vi "Dashboard Main.vi"() -> ()   [LabVIEW 2014]
uses:
  <vilib>/event_ctls.llb/eventvkey.ctl
  <vilib>/Rock Robotics/WPI/Dashboard/WPI_DashboardLogging Global.vi
  <vilib>/Rock Robotics/Network Tables/SD Read Boolean.vi
  <vilib>/Rock Robotics/Network Tables/SD Read Number.vi
  <vilib>/Utility/config.llb/Write Key (String).vi
  <vilib>/Utility/config.llb/Write Key (I32).vi
  <vilib>/Utility/config.llb/NI_LVConfig.lvlib
panel:
  in  "TCP":refnum<k5>
  in  "Rec Mode":enum32{"Stop", "Record", "Playback"}(radio)
  in  "Vision":u16(ring) items=["Camera Off", "USB Camera SW", "USB Camera HW", "IP Camera"]
  out "Camera IP":string
  out "Image Message":string="Timeout in Camera Communications"
  in  "Dashboard Tab":T1(tab)
  in  "Camera Settings":T2={"Frame Rate"=30, "Compression"=30, "Size"=1} {"Frame Rate" scale=1.0..30.0; "Size" items=["640x480", "320x240", "160x120"]}
  out "MotorChart R":cluster{"Numeric":dbl, "Numeric":dbl}(graph)
  out "MotorChart L":T3(graph)
  out "MotorSliders R":cluster{"MotorSlide1":dbl, "MotorSlide2":dbl} {"MotorSlide2" scale=-1.0..1.0 scale format="%#_2e"; "MotorSlide1" scale=-1.0..1.0 scale format="%#_2e"}
  out "MotorSliders L":T4 {"MotorSlide4 2" scale=0.0..14.0 scale format="%#_2e"; "MotorSlide2" scale=-1.0..1.0 scale format="%#_2e"; "MotorSlide1" scale=-1.0..1.0 scale format="%#_2e"}
  out "Gyro":dbl(knob) scale=0.0..360.0
  out "JS1 Z":dbl(slide) scale=-1.0..1.0 scale format="%#_2e"
  out "JS1 Graph":cluster{"X":dbl, "Y":dbl}[](graph)
  out "JS1 Buttons":T5
  out "JS2 Z":dbl(slide) scale=-1.0..1.0 scale format="%#_2e"
  out "JS2 Graph":cluster{"X":dbl, "Y":dbl}[](graph)
  out "JS2 Buttons":T5
  out "Mode":T6(ring)=enum."Auto Disabled"
  in  "DB Camera Config":bool
  out "fps":dbl format="%#.1g"
  out "Mbps":dbl format="%#.1g"
  out "Mbps 2":bool
  in  "DB/String 9":string
  in  "DB/String 8":string
  in  "DB/String 7":string
  in  "DB/String 6":string
  in  "DB/String 5":string
  in  "DB/String 4":string
  in  "DB/String 3":string
  in  "DB/String 2":string
  in  "DB/String 1":string
  in  "DB/String 0":string
  in  "DB/Slider 0":dbl(slide) scale=0.0..5.0
  in  "DB/Slider 1":dbl(slide) scale=0.0..5.0
  in  "DB/Slider 2":dbl(slide) scale=0.0..5.0
  in  "DB/Slider 3":dbl(slide) scale=0.0..5.0
  out "DB/LED 3":bool
  out "DB/LED 2":bool
  out "DB/LED 1":bool
  out "DB/LED 0":bool
  in  "DB/Button 3":bool
  in  "DB/Button 2":bool
  in  "DB/Button 1":bool
  in  "DB/Button 0":bool caption="New Name"
  out "Lifting Arm Mode":bool
  out "Lifting Arm Direction":bool
  out "Lifting Motor Speed":dbl(knob) scale=-1.0..1.0
  out "Lower Switch":bool
  out "Upper Switch":bool
  out "Auto 3":bool
  out "Auto 2":bool
  out "Auto 4":bool
  out "Auto 1":bool
  out "Lifting Arm Running":bool
  out "Trigger Switch Activated":bool
  out "Stopper Motor Speed":dbl(knob) scale=-1.0..1.0
  in  "Test Slider":dbl(slide) scale=0.0..100.0 scale format="%#_3g"
  in  "On/Off":bool caption="Solenoid"
  in  "Test Name":u16(ring) items=["Select the test to run...", "Example Test", "-------------------------------", "List of tests is built in robot code.", "Replace with your own automated tests."]
  in  "Test Tree":string(tree)
  in  "Motor":cluster{"Value":dbl, "Enable":bool} {"Value" scale=-1.0..1.0 scale format="%#_3g"}
  out "Progress":T7 {"Test Progress" scale=0.0..100.0}
  in  "Rev/Fwd":cluster{"Forward":bool, "Reverse":bool}
  in  "Test Ring":u16(ring) items=["Monochrome", "Color"]
  in  "Listbox":i32(listbox)
  out "Tree":string(tree)
  out "Camera Image":T8(plugin-control)
  out "Boolean":bool
  # "Left"
  # "Front"
  # "Right"
  # "Battery"
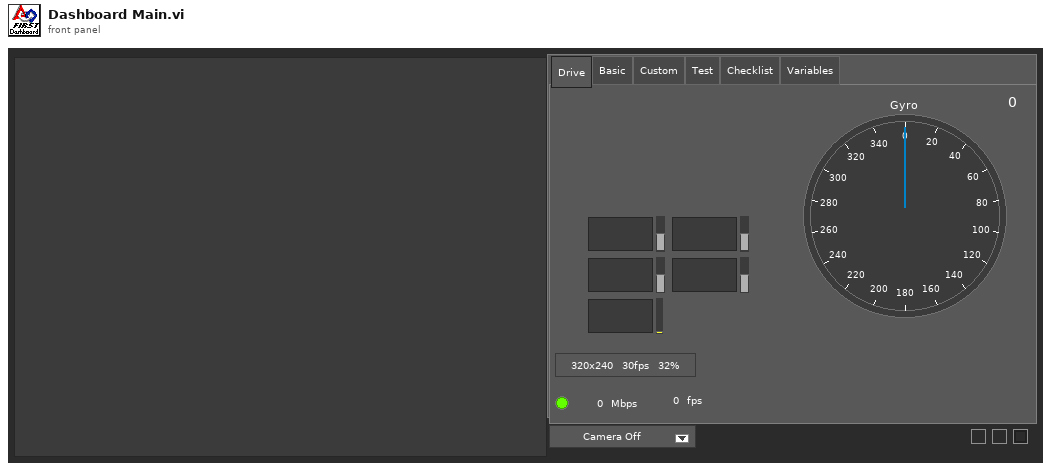
[diagram p1: front panel]
types:
  T1 = enum32{"Drive", "Basic", "Custom", "Test", "Checklist", "Variables"}
  T2 = cluster{"Frame Rate":i32, "Compression":i32, "Size":u16}
  T3 = cluster{"Numeric":dbl, "Numeric":dbl, "Battery V":dbl}
  T4 = cluster{"MotorSlide1":dbl, "MotorSlide2":dbl, "MotorSlide4 2":dbl}
  T5 = cluster{bool, bool, bool, bool, bool, bool, bool, bool, bool, bool, bool, bool}
  T6 = enum8{"Tele-Op Disabled", "Tele-Op Enabled", "Auto Disabled", "Auto Enabled", "Test Disabled", "Test Enabled", "Disconnected", "No Code", "E-Stop"}
  T7 = cluster{"Test Progress":u8, "Test Progress Text":string}
  T8 = typedef "IMAQ Image.ctl" = refnum<image>
  T9 = typedef "Image Type" = u32
  T10 = cluster{"Camera Image":refnum<vi>, "Dashboard Tab":refnum<vi>, "Boolean":refnum<vi>, "Vision":refnum<vi>, "Rec Mode":refnum<vi>, "Test Slider":refnum<vi>, "On/Off ":refnum<vi>, "Test Ring":refnum<vi>, "Rev/Fwd":refnum<vi>, "Test Name":refnum<vi>, "Motor":refnum<vi>, "Progress":refnum<vi>, "CheckList":refnum<vi>, "Tree":refnum<vi>, "Test Tree":refnum<vi>}
  T11 = cluster{"Error Strings":string, "Disable Counts":cluster{u16, u16}, "Rail Faults":cluster{u16, u16, u16}, "Robot IP":string, "DB Mode":u8, "Event Info":cluster{"Name":string, "Type":u8, "Number":u16, "Replay":u8}, "Camera Addr":string}
  T12 = cluster{"Storage":cluster{"Disk Free":u64, "RAM Block":u32, "RAM free":u32}, "CPU Utilization":cluster{"CPU % ISR":sgl, "CPU % Time Crit":sgl, "CPU % Timed Str":sgl, "CPU % High":sgl, "CPU % Above":sgl, "CPU % Normal":sgl, "CPU % Low":sgl}, "CAN":cluster{"% Bus Utilization":sgl, "Bus Off Cnt":u32, "TX_FIFO Full Cnt":u32, "Receive Error Cnt":u8, "Transmit Error Cnt":u8}, "HID":cluster{"HID Outputs":u32, "Rumble Low":u16, "Rumble High":u16}[]}
  T13 = cluster{"Status bits":cluster{"Test Mode":bool, "Autonomous":bool, "Enabled":bool, "Code Start":bool, "Brownout":bool, "Reserved 2":bool, "Reserved 3":bool, "E-Stop":bool}, "Code Trace":cluster{"Disabled":bool, "TeleOp":bool, "Auto":bool, "Test":bool}, "Controller Type":enum16{"unknown", "cRIO", "roboRio"}, "Code?":enum16{"unknown", "noCode", "code"}, "Battery V":dbl}
  T14 = cluster{"Control Bits":cluster{"TestMode":bool, "Autonomous":bool, "Enabled":bool, "FMS Present":bool, bool, bool, bool, "E-Stop":bool}, "Team Station ":u8, "Countdown":sgl, "Joystick Values":cluster{"Axes":dbl[], "Buttons":bool[], "POVs":i16[]}[]}
  T15 = cluster{"Axes":dbl[], "Buttons":bool[], "POVs":i16[]}[]
  T16 = cluster{"Axes":dbl[], "Buttons":bool[], "POVs":i16[]}
  T17 = cluster{"Buttons[0]":bool, "Buttons[1]":bool, "Buttons[2]":bool, "Buttons[3]":bool, "Buttons[4]":bool, "Buttons[5]":bool, "Buttons[6]":bool, "Buttons[7]":bool, "Buttons[8]":bool, "Buttons[9]":bool, "Buttons[10]":bool, "Buttons[11]":bool}
  T18 = typedef "NI_LVConfig.lvlib/Config Data RefNum.ctl" = refnum<k1>
  T19 = cluster{"Operation":enum16{"Update", "Clear"}, "Color Box":u32}[]
  T20 = typedef "eventvkey.ctl" = enum16{"ASCII", "Enter", "Return", "Shift", "Ctrl", "Alt", "Cmd", "Opt", "Caps", "NumLock", "Clear", "Break", "Up", "Down", "Left", "Right", "Insert", "Delete", "Home", "End", "PageUp", "PageDown", "Escape", "Help", "Pause", "ScrollLock", "F1", "F2", "F3", "F4", "F5", "F6", "F7", "F8", "F9", "F10", "F11", "F12", "F13", "F14", "F15", "F16", "F17", "F18", "F19", "F20", "F21", "F22", "F23", "F24", "Play", "VolumeUp", "VolumeDown", "Mute", "Two Byte Char"}
  T21 = cluster{"Image Size":bool, "Image Type":bool, "Pixel Value":bool, "ROI Information":bool, "Zoom Factor":bool}
  T22 = enum8{"Enabled", "Disabled", "Disabled and Grayed Out"}
  T23 = cluster{"Operation":enum16{"Update", "Clear"}, "Color Box":u32}
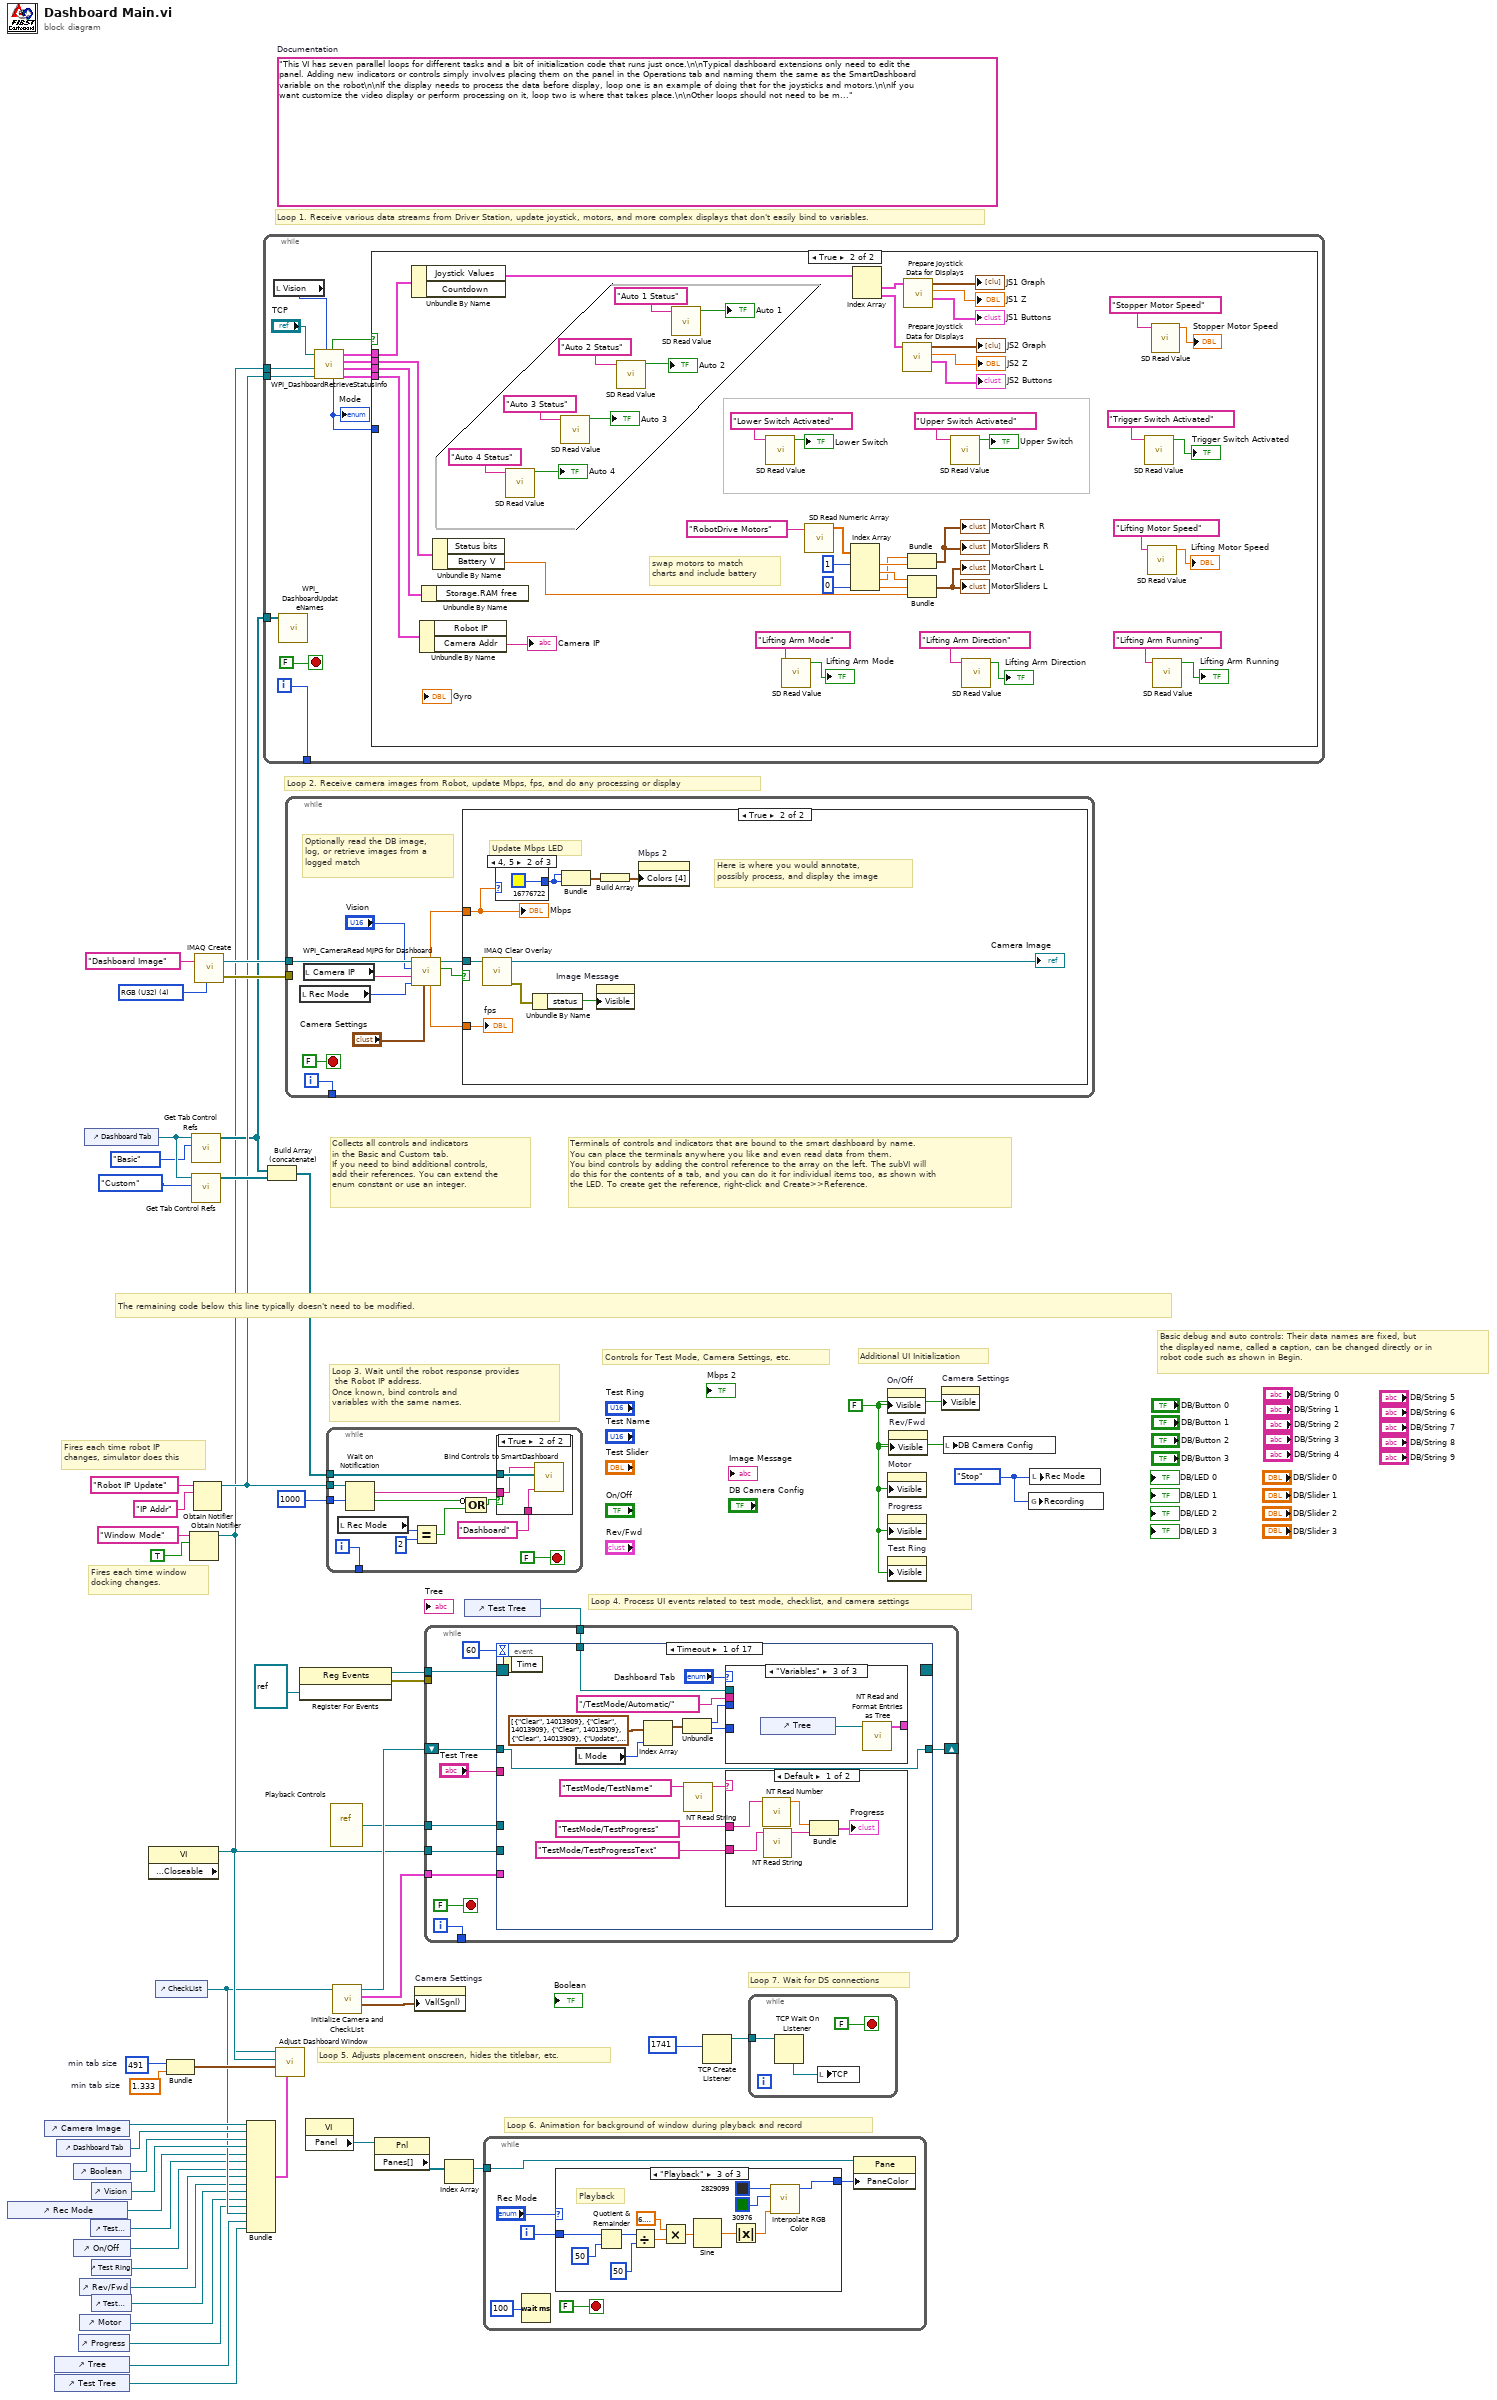
[diagram p0: block diagram]
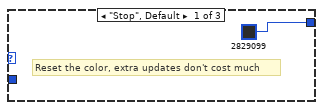
[diagram p3: hidden frame]
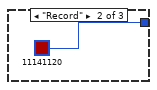
[diagram p4: hidden frame]
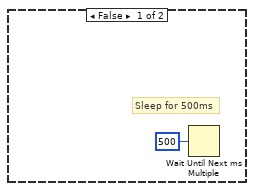
[diagram p6: hidden frame]
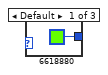
[diagram p7: hidden frame]
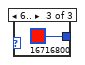
[diagram p8: hidden frame]
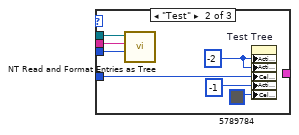
[diagram p10: hidden frame]
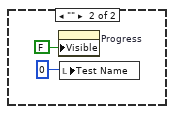
[diagram p11: hidden frame]
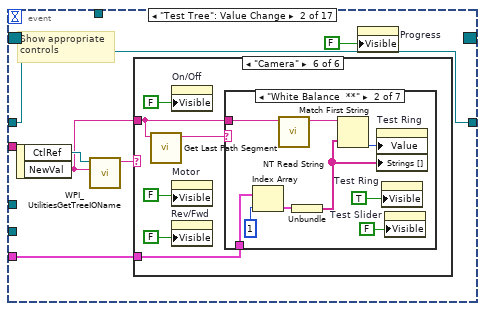
[diagram p12: hidden frame]
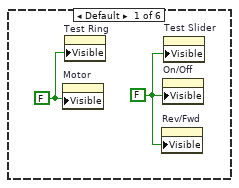
[diagram p13: hidden frame]
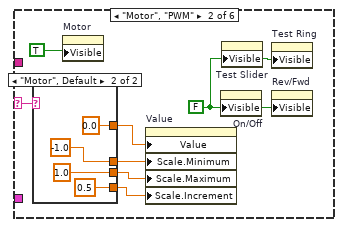
[diagram p14: hidden frame]
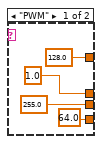
[diagram p15: hidden frame]
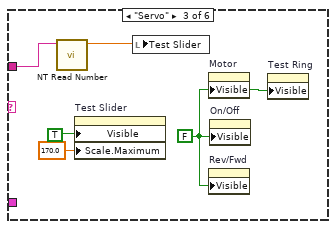
[diagram p16: hidden frame]
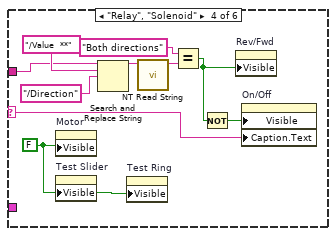
[diagram p17: hidden frame]
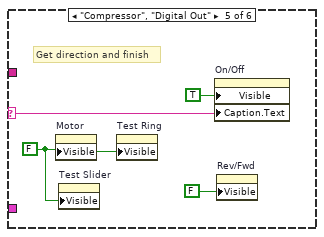
[diagram p18: hidden frame]
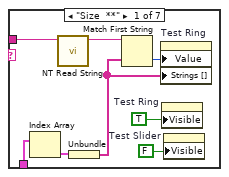
[diagram p19: hidden frame]
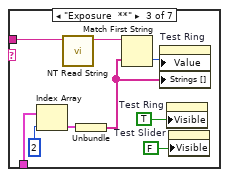
[diagram p20: hidden frame]
diagram:
  w24 = 491  # min tab size
  w23 = 1.333  # min tab size
  w32 = enum32{"Stop", "Record", "Playback"}."Stop" ("Rec Mode")
  w6 = FALSE ("Visible")
  (unwired) "This VI has seven parallel loops for different tasks and a bit of initialization code that runs just once.\n\nTypical dashboard extensions only need to edit the panel. Adding new indicators or controls simply involves placing them on the panel in the Operations tab and naming them the same as the SmartDashboard variable on the robot\n\nIf the display needs to process the data before display, loop one is an example of doing that for the joysticks and motors.\n\nIf you want customize the video display or perform processing on it, loop two is where that takes place.\n\nOther loops should not need to be modified. They are pretty standard, and document the task they perform."  # Documentation
  w52 = T9 4 items=["Grayscale (U8)", "Grayscale (I16)", "Grayscale (SGL)", "Complex (CSG)", "RGB (U32)", "HSL (U32)", "RGB (U64)"] ("Image Type")
  # "Loop 7. Wait for DS connections"
  # "Basic debug and auto controls: Their data names are fixed, but\nthe displayed name, called a caption, can be changed directly or in\nrobot code such as shown in Begin."
  # "Controls for Test Mode, Camera Settings, etc."
  # "Additional UI Initialization"
  # "Loop 6. Animation for background of window during playback and record"
  # "Fires each time robot IP\nchanges, simulator does this"
  # "Fires each time window\ndocking changes."
  # "Collects all controls and indicators\nin the Basic and Custom tab.\nIf you need to bind additional controls,\nadd their references. You can extend the\nenum constant or use an integer."
  # "The remaining code below this line typically doesn't need to be modified."
  # "Loop 4. Process UI events related to test mode, checklist, and camera settings"
  # "Terminals of controls and indicators that are bound to the smart dashboard by name.\nYou can place the terminals anywhere you like and even read data from them.\nYou bind controls by adding the control reference to the array on the left. The subVI will\ndo this for the contents of a tab, and you can do it for individual items too, as shown with\nthe LED. To create get the reference, right-click and Create>>Reference."
  # "Loop 3. Wait until the robot response provides\n the Robot IP address.\nOnce known, bind controls and\nvariables with the same names."
  # "Loop 5. Adjusts placement onscreen, hides the titlebar, etc."
  # "Loop 1. Receive various data streams from Driver Station, update joystick, motors, and more complex displays that don't easily bind to variables."
  # "Loop 2. Receive camera images from Robot, update Mbps, fps, and do any processing or display"
  n1 = control-ref of="Rec Mode"() -> (w12:refnum<vi>)
  n2 = control-ref of="Camera Image"() -> (w27:refnum<vi>)
  n3 = control-ref of="Tree"() -> (w16:refnum<vi>)
  n4 = control-ref of="Test Tree"() -> (w15:refnum<vi>)
  n5 = control-ref of="Dashboard Tab"() -> (w26:refnum<vi>)
  n6 = control-ref of="Boolean"() -> (w21:refnum<vi>)
  n7 = control-ref of="On/Off"() -> (w10:refnum<vi>)
  n8 = control-ref of="Progress"() -> (w7:refnum<vi>)
  n9 = control-ref of="Rev/Fwd"() -> (w8:refnum<vi>)
  n10 = control-ref of="Motor"() -> (w13:refnum<vi>)
  n11 = control-ref of="Dashboard Tab"() -> (w30:refnum<vi>)
  n12 = control-ref of="Test Slider"() -> (w11:refnum<vi>)
  n13 = control-ref of="Vision"() -> (w25:refnum<vi>)
  n14 = control-ref of="Test Ring"() -> (w9:refnum<vi>)
  n15 = control-ref of="Test Name"() -> (w14:refnum<vi>)
  n16 = property class="VI" props=["Front Panel.Closeable"]() -> (reference out=w31:refnum<vi>)  [unwired: 2 in, 2 out]
  n17 = control-ref of="CheckList"() -> (w17:refnum<vi>)
  n18 = Bundle("min tab size"=w24, "min tab size"=w23) -> (w22:cluster{"min tab size":i32, "min tab size":dbl})  [unwired: 1 in]
  n19 = Obtain Notifier(name (unnamed)="Window Mode", notification data type=TRUE) -> (notifier out=w3:refnum<notifier>)  [unwired: 2 in, 2 out]
  n20 = call <vilib>:"Get Tab Control Refs.vi"("Page Index"=T1."Basic" ("Dashboard Tab"), "TabControl in"=w30) -> ("ControlsOnPage"=w4:refnum<vi>[])  [unwired: 9 in]
  n21 = call <vilib>:"Get Tab Control Refs.vi"("Page Index"=T1."Custom" ("Dashboard Tab"), "TabControl in"=w30) -> ("ControlsOnPage"=w29:refnum<vi>[])  [unwired: 9 in]
  n22 = Obtain Notifier(name (unnamed)="Robot IP Update", notification data type="IP Addr" ("name (unnamed)")) -> (notifier out=w5:refnum<notifier>)  [unwired: 2 in, 2 out]
  n23 = call "IMAQ Create"("Image Name"="Dashboard Image", "Image Type"=w52) -> ("New Image"=w50:T8, "error out"=w49:errorcluster)  [unwired: 2 in, 1 out]
  n24 = Bundle("Camera Image"=w27, "Dashboard Tab"=w26, "Boolean"=w21, "Vision"=w25, "Rec Mode"=w12, "Test Slider"=w11, "On/Off"=w10, "Test Ring"=w9, "Rev/Fwd"=w8, "Test Name"=w14, "Motor"=w13, "Progress"=w7, "CheckList"=w17, "Tree"=w16, "Test Tree"=w15) -> (w18:T10)  [unwired: 1 in]
  n25 = while {
    tunnel: [w64] -> _
    tunnel: w5 -> [w58]
    tunnel: w4 -> [w57]
    tunnel: w3 -> [w53]
    i -> [w64]
    stop <- FALSE stop-if-true
    n26 = local read "Vision"() -> (w55:u16)
    n27 = call <vilib>:"WPI_DashboardUpdateNames.vi"("Controls on Tab"=w57) -> ()  [unwired: 11 in]
    n28 = call <vilib>:"WPI_DashboardRetrieveStatusInfo.vi"("Vision"=w55, "Binding Refnum"=w58, "Window Mode Notifier"=w53, "TCP Cnx"="TCP") -> ("Power and Errors"=w59:T11, "Robot Metrics"=w62:T12, "Status Info"=w63:T13, "Control Info"=w60:T14, "Robot Mode"=w56:T6, "Process?"=w61:bool)  [unwired: 2 in]
    "Mode" <- w56
    n29 = case shown="True" w61 {
      tunnel: w63 -> [_ w114]
      tunnel: w62 -> [_ w113]
      tunnel: w60 -> [_ w112]
      tunnel: w59 -> [_ w111]
      tunnel: w56 -> [_ _]
      frame False {
      }
      frame True {
        # "swap motors to match\ncharts and include battery"
        n30 = Unbundle By Name(w112) -> ("Joystick Values"=w100:T15)  [unwired: 1 out]
        n31 = Unbundle By Name(w111) -> ("Camera Addr"=→"Camera IP":string)  [unwired: 1 out]
        n32 = Unbundle By Name(w113) -> ()  [unwired: 1 out]
        n33 = Unbundle By Name(w114) -> ("Battery V"=w78:dbl)  [unwired: 1 out]
        n34 = call-poly <vilib>:"SD Read Value.vi"("Name"="Auto 4 Status") -> ("Boolean"=→"Auto 4":bool)  [unwired: 8 in, 2 out]
        n35 = call-poly <vilib>:"SD Read Value.vi"("Name"="Auto 3 Status") -> ("Boolean"=→"Auto 3":bool)  [unwired: 8 in, 2 out]
        n36 = call-poly <vilib>:"SD Read Value.vi"("Name"="Auto 2 Status") -> ("Boolean"=→"Auto 2":bool)  [unwired: 8 in, 2 out]
        n37 = call-poly <vilib>:"SD Read Value.vi"("Name"="Auto 1 Status") -> ("Boolean"=→"Auto 1":bool)  [unwired: 8 in, 2 out]
        n38 = call-poly <vilib>:"SD Read Value.vi"("Name"="Lower Switch Activated") -> ("Boolean"=→"Lower Switch":bool)  [unwired: 8 in, 2 out]
        n39 = call-poly <vilib>:"SD Read Value.vi"("Name"="Lifting Arm Mode" ("refnum name")) -> ("Boolean"=→"Lifting Arm Mode":bool)  [unwired: 8 in, 2 out]
        n40 = call <vilib>:"SD Read Numeric Array.vi"("Name"="RobotDrive Motors") -> ("Numeric Array"=w102:dbl[])  [unwired: 8 in, 2 out]
        n41 = Index Array(array=w102, index #1=1, index #4=0) -> (element #1=w106:dbl, element #2=w107:dbl, element #3=w105:dbl, element #4=w110:dbl)  [unwired: 2 in]
        n42 = Index Array(array=w100) -> (element #1=w99:T16, element #2=w94:T16)  [unwired: 2 in]
        n43 = call "Prepare Joystick Data for Displays.vi"("Joystick Values"=w94) -> ("Buttons"=→"JS2 Buttons":T17, "Z Axis"=→"JS2 Z":dbl, "Cartesian Data"=→"JS2 Graph":cluster{"X axis":dbl, "X axis":dbl}[])  [unwired: 8 in]
        n44 = call "Prepare Joystick Data for Displays.vi"("Joystick Values"=w99) -> ("Buttons"=→"JS1 Buttons":T17, "Z Axis"=→"JS1 Z":dbl, "Cartesian Data"=→"JS1 Graph":cluster{"X axis":dbl, "X axis":dbl}[])  [unwired: 8 in]
        n45 = Bundle("Numeric"=w105, "Numeric"=w106) -> (→"MotorChart R" →"MotorSliders R":cluster{"Numeric":dbl, "Numeric":dbl})  [unwired: 1 in]
        n46 = Bundle("Numeric"=w107, "Numeric"=w110, "Battery V"=w78) -> (→"MotorChart L" →"MotorSliders L":T3)  [unwired: 1 in]
        n47 = call-poly <vilib>:"SD Read Value.vi"("Name"="Upper Switch Activated") -> ("Boolean"=→"Upper Switch":bool)  [unwired: 8 in, 2 out]
        n48 = call-poly <vilib>:"SD Read Value.vi"("Name"="Lifting Arm Direction" ("refnum name")) -> ("Boolean"=→"Lifting Arm Direction":bool)  [unwired: 8 in, 2 out]
        n49 = call-poly <vilib>:"SD Read Value.vi"("Name"="Trigger Switch Activated" ("refnum name")) -> ("Boolean"=→"Trigger Switch Activated":bool)  [unwired: 8 in, 2 out]
        n50 = call-poly <vilib>:"SD Read Value.vi"("Name"="Lifting Motor Speed" ("refnum name")) -> ("Numeric"=→"Lifting Motor Speed":dbl)  [unwired: 8 in, 2 out]
        n51 = call-poly <vilib>:"SD Read Value.vi"("Name"="Stopper Motor Speed" ("refnum name")) -> ("Numeric"=→"Stopper Motor Speed":dbl)  [unwired: 8 in, 2 out]
        n52 = call-poly <vilib>:"SD Read Value.vi"("Name"="Lifting Arm Running" ("refnum name")) -> ("Boolean"=→"Lifting Arm Running":bool)  [unwired: 8 in, 2 out]
      }
    }
  }
  n53 = Build Array (concatenate)(w4, w29) -> (w28:refnum<vi>[])
  n54 = call "Adjust Dashboard Window.vi"("Sizing Refnums"=w18, "Size Constraints"=w22, "VI"=w31, "Notifier in"=w3) -> ()  [unwired: 8 in]
  n55 = while {
    tunnel: w50 -> [w123]
    tunnel: w49 -> [_]
    tunnel: [w124] -> _
    i -> [w124]
    stop <- FALSE stop-if-true
    # "Optionally read the DB image,\nlog, or retrieve images from a\nlogged match"
    n56 = local read "Rec Mode"() -> (w117:enum32{"Stop", "Record", "Playback"})
    n57 = local read "Camera IP"() -> (w115:string)
    n58 = call <vilib>:"WPI_CameraRead MJPG for Dashboard.vi"("Camera Settings"="Camera Settings", "Rec Mode"=w117, "Camera IP"=w115, "Camera Mode"="Vision", "Refnum in"=w123) -> ("Active"=w121:bool, "Refnum out"=w122:T8, "FPS"=w120:dbl, "Bandwidth (Mbps)"=w119:dbl)  [unwired: 3 in]
    n59 = case shown="True" w121 {
      tunnel: w122 -> [_ w130]
      tunnel: w119 -> [_ w129]
      tunnel: w120 -> [_ w127]
      frame False {
        # "Sleep for 500ms"
        n60 = Wait Until Next ms Multiple(millisecond multiple=u32 500) -> ()  [unwired: 1 out]
      }
      frame True {
        # "Here is where you would annotate,\npossibly process, and display the image"
        # "Update Mbps LED"
        n61 = call "IMAQ Clear Overlay"("Image"=w130) -> ("error out"=w134:errorcluster, "Image Out"=→"Camera Image":T8)  [unwired: 2 in, 7 out]
        n62 = case shown="4, 5" w129 {
          tunnel: [u32 6618880 ("Color Box") u32 16776722 ("Color Box") u32 16716800 ("Color Box")] -> w131
          frame Default {
          }
          frame 4, 5 {
          }
          frame 6.. {
          }
        }
        n63 = Unbundle By Name(w134) -> ("status"=w135:bool)
        n64 = Bundle("Color Box"=w131, "Color Box"=w131) -> (w133:cluster{"Color Box":u32, "Color Box":u32})  [unwired: 1 out]
        n65 = property on="Image Message" class="Str"("Visible"=w135) -> ()  [unwired: 2 in, 2 out]
        n66 = Build Array(w133) -> (w132:cluster{"Color Box":u32, "Color Box":u32}[])
        n67 = property on="Mbps 2" class="Bool (strict)"("Colors [4]"=w132) -> ()  [unwired: 2 in, 2 out]
        "Mbps" <- w129
        "fps" <- w127
      }
    }
  }
  n68 = register-events(refnum<vi> refnum) -> (reference out=w36:refnum<event-registration>, error out=w35:errorcluster)  [unwired: 2 in]
  n69 = property class="VI"() -> ("Panel"=w39:refnum<vi>)  [unwired: 2 in, 2 out]
  n70 = while {
    tunnel: w28 -> [w150]
    tunnel: w5 -> [w148]
    tunnel: [w146] -> _
    tunnel: u32 1000 ("milliseconds to wait") -> [w145]
    i -> [w146]
    stop <- FALSE stop-if-true
    n71 = local read "Rec Mode"() -> (w141:enum32{"Stop", "Record", "Playback"})
    n72 = Wait on Notification(notifier=w148, timeout in ms (-1)=w145) -> (notification=w147:string, timed out?=w143:bool)  [unwired: 2 in, 2 out]
    n73 = Equal?(x=w141, y=u16 2 ("Rec Mode")) -> (x = y?=w142:bool)
    n74 = Compound Arithmetic op=OR(invert w143, w142) -> (w144:bool)
    n75 = case shown="True" w144 {
      tunnel: w150 -> [_ w153]
      tunnel: w147 -> [_ w152]
      tunnel: "Dashboard" -> [_ w151]
      frame False {
      }
      frame True {
        n76 = call <vilib>:"Bind Controls to SmartDashboard.vi"("Client Name"=w151, "Bound Control Refs"=w153, "Server IP Address"=w152) -> ()  [unwired: 9 in]
      }
    }
  }
  n77 = vi-ref "Playback Controls.vi"() -> (w37:refnum<vi>)
  n78 = call "Initialize Camera and CheckList.vi"("ListBox in"=w17) -> ("Cluster"=w43:cluster{"value":i32, "value":i32, "index":i32}, "Array"=w44:cluster{string[]}[], "File Refnum"=w42:T18)  [unwired: 8 in]
  n79 = property class="Pnl"(reference=w39) -> ("Panes[]"=w40:refnum<vi>[])  [unwired: 1 in, 2 out]
  n80 = property on="Camera Settings" class="Clust (strict)"("Val(Sgnl)"=w43) -> ()  [unwired: 2 in, 2 out]
  n81 = Index Array(array=w40) -> (element=w38:refnum<vi>)  [unwired: 1 in]
  n82 = control-ref of="Test Tree"() -> (w41:refnum<vi>)
  n83 = while {
    tunnel: w44 -> [w161]
    shift-right: [w160] -> _
    shift-left: w42 -> [w159]
    tunnel: [w158] -> _
    tunnel: w41 -> [w157]
    tunnel: w37 -> [w156]
    tunnel: w36 -> [w155]
    tunnel: w35 -> [_]
    tunnel: w31 -> [w154]
    i -> [w158]
    stop <- FALSE stop-if-true
    n84 = event shown="[0] Timeout" {
      selector: w155 -> [_ _ _ _ _ _ _ _ _ _ _ _ _ _ _ _ _]
      dyn-events: [_ _ _ _ _ _ _ _ _ _ _ _ _ w399 _ _ _] -> _
      timeout: u32 60 ("milliseconds to wait") -> [_ _ _ _ _ _ _ _ _ _ _ _ _ _ _ _ _]
      tunnel: w157 -> [w173 _ _ _ _ _ _ _ _ _ _ _ _ _ _ _ _]
      tunnel: "Test Tree" -> [_ _ _ _ _ _ _ _ w368 w376 w378 w382 w390 _ _ _ _]
      tunnel: w161 -> [_ w195 _ _ _ _ w332 w362 _ _ _ _ _ _ _ _ _]
      tunnel: [w169 w194 w293 w298 w306 w318 w331 w355 w367 w374 w377 w381 w389 w401 w415 w416 w426] -> w160
      tunnel: w159 -> [w169 w194 w293 w298 w306 w318 w330 w355 w367 w374 w377 w381 w389 w401 w415 w416 w426]
      tunnel: w156 -> [_ _ _ _ _ _ _ _ _ _ _ _ _ w402 _ w419 _]
      tunnel: w154 -> [_ _ _ _ _ _ _ _ _ _ _ _ _ w397 _ _ _]
      event Timeout {
        n85 = event-data() -> ()  [unwired: 1 in, 1 out]
        n86 = local read "Mode"() -> (w172:T6)
        n87 = Index Array(array=T19 [{"Operation"=enum."Clear", "Color Box"=14013909}, {"Operation"=enum."Clear", "Color Box"=14013909}, {"Operation"=enum."Clear", "Color Box"=14013909}, {"Operation"=enum."Clear", "Color Box"=14013909}, {"Operation"=enum."Update", "Color Box"=14013909}, {"Operation"=enum."Update", "Color Box"=16777215}, {"Operation"=enum."Clear", "Color Box"=14013909}, {"Operation"=enum."Clear", "Color Box"=14013909}, {"Operation"=enum."Clear", "Color Box"=14013909}], index=w172) -> (element=w167:T23)
        n88 = Unbundle(w167) -> ("Operation"=w166:enum16{"Update", "Clear"}, "Color Box"=w165:u32)
        n89 = call <vilib>:"NT Read String.vi"("Name"="TestMode/TestName") -> ("String"=w176:string)  [unwired: 9 in, 1 out]
        n90 = case shown="\"Variables\"" "Dashboard Tab" {
          tunnel: w173 -> [_ w184 _]
          tunnel: "/TestMode/Automatic/" ("Name Pattern") -> [_ w183 _]
          tunnel: w166 -> [_ w182 _]
          tunnel: [_ _ w186] -> _
          tunnel: w165 -> [_ w178 _]
          frame "Custom", Default {
          }
          frame "Test" {
            w181 = -2 ("Active Item:Row Number")
            n91 = call <vilib>:"NT Read and Format Entries as Tree.vi"("Operation"=w182, "Name Pattern"=w183, "Tree Refnum"=w184) -> ()  [unwired: 7 in, 2 out]
            n92 = property on="Test Tree" class="Tree (strict)"("Active Item Row Number"=w181, "ActiveColNum"=w181, "CellBG"=w178, "Active Item Row Number"=-1 ("Active Item:Row Number"), "CellBG"=u32 5789784 ("Color Box")) -> ()  [unwired: 2 in, 2 out]
          }
          frame "Variables" {
            n93 = control-ref of="Tree"() -> (w185:refnum<vi>)
            n94 = call <vilib>:"NT Read and Format Entries as Tree.vi"("Tree Refnum"=w185) -> ("Formatted Strings"=w186:cluster{"Name":string, "Value":string}[])  [unwired: 9 in, 1 out]
          }
        }
        n95 = case shown="Default" w176 {
          tunnel: "TestMode/TestProgress" ("Name") -> [w188 _]
          tunnel: "TestMode/TestProgressText" ("Name") -> [w187 _]
          frame Default {
            n96 = call <vilib>:"NT Read Number.vi"("Name"=w188) -> ("Numeric"=w189:dbl)  [unwired: 9 in, 1 out]
            n97 = call <vilib>:"NT Read String.vi"("Name"=w187) -> ("String"=w190:string)  [unwired: 9 in, 1 out]
            n98 = Bundle("Numeric"=w189, "String"=w190) -> (→"Progress":cluster{"Numeric":dbl, "String":string})  [unwired: 1 in]
          }
          frame "" {
            n99 = property on="Progress" class="Clust (strict)"("Visible"=FALSE) -> ()  [unwired: 2 in, 2 out]
            n100 = local write "Test Name"(u16 0) -> ()
          }
        }
      }
      event "Test Tree": Value Change {
        # "Show appropriate\ncontrols"
        n101 = event-data() -> ("CtlRef"=w198:refnum<vi>, "NewVal"=w196:string)  [unwired: 1 in]
        n102 = call <vilib>:"WPI_UtilitiesGetTreeIOName.vi"("NewVal"=w196, "TreeControl in"=w198) -> ("I/O Name"=w199:string)  [unwired: 9 in]
        n103 = case shown="\"Camera\"" w199 {
          selector: w199 -> [_ w206 _ w224 w233 _]
          tunnel: w196 -> [_ _ w221 w223 _ w240]
          tunnel: w195 -> [_ _ _ _ _ w239]
          frame Default {
            w201 = FALSE ("Visible")
            w200 = FALSE ("Visible")
            n104 = property on="Motor" class="Clust (strict)"("Visible"=w200) -> ()  [unwired: 2 in, 2 out]
            n105 = property on="Test Ring" class="Ring (strict)"("Visible"=w200) -> ()  [unwired: 2 in, 2 out]
            n106 = property on="Rev/Fwd" class="Clust (strict)"("Visible"=w201) -> ()  [unwired: 2 in, 2 out]
            n107 = property on="On/Off" class="Bool (strict)"("Visible"=w201) -> ()  [unwired: 2 in, 2 out]
            n108 = property on="Test Slider" class="Slide (strict)"("Visible"=w201) -> ()  [unwired: 2 in, 2 out]
          }
          frame "Motor", "PWM" {
            w207 = FALSE ("Visible")
            n109 = case shown="\"Motor\", Default" w206 {
              tunnel: [1.0 ("Value") -1.0 ("Value")] -> w205
              tunnel: [255.0 ("Value") 1.0 ("Value")] -> w204
              tunnel: [128.0 ("Value") 0.0 ("Value")] -> w203
              tunnel: [64.0 ("Value") 0.5 ("Value")] -> w202
              frame "PWM" {
              }
              frame "Motor", Default {
              }
            }
            n110 = property on="Motor" class="Clust (strict)"("Visible"=TRUE) -> ()  [unwired: 2 in, 2 out]
            n111 = property on="Value" class="Slide (strict)"("Value"=w203, "Scale.Minimum"=w205, "Scale.Maximum"=w204, "Scale.Increment"=w202) -> ()  [unwired: 2 in, 2 out]
            n112 = property on="On/Off" class="Bool (strict)"("Visible"=w207) -> ()  [unwired: 2 in, 2 out]
            n113 = property on="Test Slider" class="Slide (strict)"("Visible"=w207) -> ()  [unwired: 2 in, 2 out]
            n114 = property on="Test Ring" class="Ring (strict)"("Visible"=w207) -> ()  [unwired: 2 in, 2 out]
            n115 = property on="Rev/Fwd" class="Clust (strict)"("Visible"=w207) -> ()  [unwired: 2 in, 2 out]
          }
          frame "Servo" {
            w219 = FALSE ("Visible")
            n116 = call <vilib>:"NT Read Number.vi"("Name"=w221) -> ("Numeric"=w220:dbl)  [unwired: 9 in, 1 out]
            n117 = property on="Test Slider" class="Slide (strict)"("Visible"=TRUE, "Scale.Maximum"=170.0 ("Scale.Range:Maximum")) -> ()  [unwired: 2 in, 2 out]
            n118 = local write "Test Slider"(w220) -> ()
            n119 = property on="Motor" class="Clust (strict)"("Visible"=w219) -> ()  [unwired: 2 in, 2 out]
            n120 = property on="Rev/Fwd" class="Clust (strict)"("Visible"=w219) -> ()  [unwired: 2 in, 2 out]
            n121 = property on="On/Off" class="Bool (strict)"("Visible"=w219) -> ()  [unwired: 2 in, 2 out]
            n122 = property on="Test Ring" class="Ring (strict)"("Visible"=w219) -> ()  [unwired: 2 in, 2 out]
          }
          frame "Relay", "Solenoid" {
            w222 = FALSE ("Visible")
            n123 = property on="Motor" class="Clust (strict)"("Visible"=w222) -> ()  [unwired: 2 in, 2 out]
            n124 = property on="Test Slider" class="Slide (strict)"("Visible"=w222) -> ()  [unwired: 2 in, 2 out]
            n125 = Search and Replace String(input string=w223, search string="/Value  **", replace string="/Direction") -> (result string=w229:string)  [unwired: 5 in, 3 out]
            n126 = property on="Test Ring" class="Ring (strict)"("Visible"=w222) -> ()  [unwired: 2 in, 2 out]
            n127 = call <vilib>:"NT Read String.vi"("Name"=w229) -> ("String"=w227:string)  [unwired: 9 in, 1 out]
            n128 = Equal?(x="Both directions", y=w227) -> (x = y?=w225:bool)
            n129 = Not(x=w225) -> (.not. x?=w226:bool)
            n130 = property on="Rev/Fwd" class="Clust (strict)"("Visible"=w225) -> ()  [unwired: 2 in, 2 out]
            n131 = property on="On/Off" class="Bool (strict)"("Visible"=w226, "Caption.Text"=w224) -> ()  [unwired: 2 in, 2 out]
          }
          frame "Compressor", "Digital Out" {
            w232 = FALSE ("Visible")
            # "Get direction and finish"
            n132 = property on="Motor" class="Clust (strict)"("Visible"=w232) -> ()  [unwired: 2 in, 2 out]
            n133 = property on="Test Slider" class="Slide (strict)"("Visible"=w232) -> ()  [unwired: 2 in, 2 out]
            n134 = property on="Test Ring" class="Ring (strict)"("Visible"=w232) -> ()  [unwired: 2 in, 2 out]
            n135 = property on="On/Off" class="Bool (strict)"("Visible"=TRUE, "Caption.Text"=w233) -> ()  [unwired: 2 in, 2 out]
            n136 = property on="Rev/Fwd" class="Clust (strict)"("Visible"=FALSE) -> ()  [unwired: 2 in, 2 out]
          }
          frame "Camera" {
            n137 = call <vilib>:"Get Last Path Segment.vi"("String in"=w240) -> ("String out"=w241:string)  [unwired: 10 in]
            n138 = property on="On/Off" class="Bool (strict)"("Visible"=FALSE) -> ()  [unwired: 2 in, 2 out]
            n139 = property on="Motor" class="Clust (strict)"("Visible"=FALSE) -> ()  [unwired: 2 in, 2 out]
            n140 = property on="Rev/Fwd" class="Clust (strict)"("Visible"=FALSE) -> ()  [unwired: 2 in, 2 out]
            n141 = case shown="\"White Balance  **\"" w241 {
              tunnel: w240 -> [w247 w256 w265 w274 w283 _ w289]
              tunnel: w239 -> [w245 w253 w262 w271 w280 _ _]
              frame "Size  **" {
                n142 = Index Array(array=w245) -> (element=w244:cluster{string[]})  [unwired: 1 in]
                n143 = call <vilib>:"NT Read String.vi"("Name"=w247) -> ("String"=w246:string)  [unwired: 9 in, 1 out]
                n144 = Unbundle(w244) -> (w242:string[])
                n145 = Match First String(2:w242, 3:w246) -> (0:w243:i32)  [unwired: 1 out]
                n146 = property on="Test Ring" class="Ring (strict)"("Value"=w243, "Strings []"=w242) -> ()  [unwired: 2 in, 2 out]
                n147 = property on="Test Ring" class="Ring (strict)"("Visible"=TRUE) -> ()  [unwired: 2 in, 2 out]
                n148 = property on="Test Slider" class="Slide (strict)"("Visible"=FALSE) -> ()  [unwired: 2 in, 2 out]
              }
              frame "White Balance  **" {
                n149 = Index Array(array=w253, index=1) -> (element=w254:cluster{string[]})
                n150 = call <vilib>:"NT Read String.vi"("Name"=w256) -> ("String"=w255:string)  [unwired: 9 in, 1 out]
                n151 = Unbundle(w254) -> (w251:string[])
                n152 = Match First String(2:w251, 3:w255) -> (0:w250:i32)  [unwired: 1 out]
                n153 = property on="Test Ring" class="Ring (strict)"("Value"=w250, "Strings []"=w251) -> ()  [unwired: 2 in, 2 out]
                n154 = property on="Test Ring" class="Ring (strict)"("Visible"=TRUE) -> ()  [unwired: 2 in, 2 out]
                n155 = property on="Test Slider" class="Slide (strict)"("Visible"=FALSE) -> ()  [unwired: 2 in, 2 out]
              }
              frame "Exposure  **" {
                n156 = Index Array(array=w262, index=2) -> (element=w263:cluster{string[]})
                n157 = call <vilib>:"NT Read String.vi"("Name"=w265) -> ("String"=w264:string)  [unwired: 9 in, 1 out]
                n158 = Unbundle(w263) -> (w259:string[])
                n159 = Match First String(2:w259, 3:w264) -> (0:w260:i32)  [unwired: 1 out]
                n160 = property on="Test Ring" class="Ring (strict)"("Value"=w260, "Strings []"=w259) -> ()  [unwired: 2 in, 2 out]
                n161 = property on="Test Ring" class="Ring (strict)"("Visible"=TRUE) -> ()  [unwired: 2 in, 2 out]
                n162 = property on="Test Slider" class="Slide (strict)"("Visible"=FALSE) -> ()  [unwired: 2 in, 2 out]
              }
              frame "Exposure Priority  **" {
                n163 = Index Array(array=w271, index=3) -> (element=w272:cluster{string[]})
                n164 = call <vilib>:"NT Read String.vi"("Name"=w274) -> ("String"=w273:string)  [unwired: 9 in, 1 out]
                n165 = Unbundle(w272) -> (w268:string[])
                n166 = Match First String(2:w268, 3:w273) -> (0:w269:i32)  [unwired: 1 out]
                n167 = property on="Test Ring" class="Ring (strict)"("Value"=w269, "Strings []"=w268) -> ()  [unwired: 2 in, 2 out]
                n168 = property on="Test Ring" class="Ring (strict)"("Visible"=TRUE) -> ()  [unwired: 2 in, 2 out]
                n169 = property on="Test Slider" class="Slide (strict)"("Visible"=FALSE) -> ()  [unwired: 2 in, 2 out]
              }
              frame "Color Enable  **" {
                n170 = Index Array(array=w280, index=4) -> (element=w281:cluster{string[]})
                n171 = call <vilib>:"NT Read String.vi"("Name"=w283) -> ("String"=w282:string)  [unwired: 9 in, 1 out]
                n172 = Unbundle(w281) -> (w277:string[])
                n173 = Match First String(2:w277, 3:w282) -> (0:w278:i32)  [unwired: 1 out]
                n174 = property on="Test Ring" class="Ring (strict)"("Value"=w278, "Strings []"=w277) -> ()  [unwired: 2 in, 2 out]
                n175 = property on="Test Ring" class="Ring (strict)"("Visible"=TRUE) -> ()  [unwired: 2 in, 2 out]
                n176 = property on="Test Slider" class="Slide (strict)"("Visible"=FALSE) -> ()  [unwired: 2 in, 2 out]
              }
              frame Default {
                n177 = property on="Test Ring" class="Ring (strict)"("Visible"=FALSE) -> ()  [unwired: 2 in, 2 out]
                n178 = property on="Test Slider" class="Slide (strict)"("Visible"=FALSE) -> ()  [unwired: 2 in, 2 out]
              }
              frame "Brightness  **", "Color Level  **", "Compression  **", "FPS  **", "Sharpness  **" {
                n179 = call <vilib>:"NT Read Number.vi"("Name"=w289) -> ("Numeric"=w288:dbl)  [unwired: 9 in, 1 out]
                n180 = local write "Test Slider"(w288) -> ()
                n181 = property on="Test Slider" class="Slide (strict)"("Visible"=TRUE, "Scale.Maximum"=100.0 ("Scale.Range:Maximum")) -> ()  [unwired: 2 in, 2 out]
                n182 = property on="Test Ring" class="Ring (strict)"("Visible"=FALSE) -> ()  [unwired: 2 in, 2 out]
              }
            }
          }
        }
        n183 = property on="Progress" class="Clust (strict)"("Visible"=FALSE) -> ()  [unwired: 2 in, 2 out]
      }
      event "Test Name": Mouse Enter {
        # "Populate the ring with the list of tests"
        n184 = event-data() -> ()  [unwired: 1 in, 1 out]
        n185 = call <vilib>:"NT Read String Array.vi"("Name"="TestMode/TestList") -> ("String Array"=w297:string[])  [unwired: 9 in, 1 out]
        n186 = Build Array (concatenate)("Select the test to run...", w297) -> (w296:string[])
        n187 = property on="Test Name" class="Ring (strict)"("Strings []"=w296) -> ()  [unwired: 2 in, 2 out]
      }
      event "Test Name": Value Change {
        w299 = FALSE ("Visible")
        # "Tell the robot the test name to run"
        n188 = event-data() -> ("NewVal"=w303:u16)  [unwired: 1 in]
        n189 = property on="Test Name" class="Ring (strict)"() -> ("Strings []"=w304:string[])  [unwired: 2 in, 2 out]
        n190 = local write "Progress"(T7 {"Test Progress"=0, "Test Progress Text"=""} ("Progress")) -> ()
        n191 = Index Array(array=w304, index=w303) -> (element=w302:string)
        n192 = call <vilib>:"NT Write String.vi"("String"=w302, "Name"="TestMode/TestName") -> ()  [unwired: 9 in, 1 out]
        n193 = property on="Progress" class="Clust (strict)"("Visible"=TRUE) -> ()  [unwired: 2 in, 2 out]
        n194 = property on="Motor" class="Clust (strict)"("Visible"=w299) -> ()  [unwired: 2 in, 2 out]
        n195 = property on="Test Slider" class="Slide (strict)"("Visible"=w299) -> ()  [unwired: 2 in, 2 out]
        n196 = property on="On/Off" class="Bool (strict)"("Visible"=w299) -> ()  [unwired: 2 in, 2 out]
        n197 = property on="Rev/Fwd" class="Clust (strict)"("Visible"=w299) -> ()  [unwired: 2 in, 2 out]
        n198 = property on="Test Ring" class="Ring (strict)"("Visible"=w299) -> ()  [unwired: 2 in, 2 out]
      }
      event "Listbox": Double Click {
        # "Shift clears all"
        # "Update symbols on the listbox"
        n199 = event-data() -> ("PlatMods.Shift"=w307:bool, "Row"=w309:i32)  [unwired: 1 in]
        n200 = case shown="True" w307 {
          tunnel: w309 -> [w313 _]
          tunnel: 1 -> [w312 _]
          frame False {
            n201 = property on="Listbox" class="LstBox (strict)"() -> ("Item Symbols"=w311:i32[])  [unwired: 2 in, 2 out]
            n202 = Replace Array Subset(array=w311, new element=w312, index=w313) -> (w310:i32[])
            n203 = property on="Listbox" class="LstBox (strict)"("Item Symbols"=w310) -> ()  [unwired: 2 in, 2 out]
          }
          frame True {
            w314 = 0 ("Top Row")
            n204 = property on="Listbox" class="LstBox (strict)"() -> ("Number of Rows"=w316:u32)  [unwired: 2 in, 2 out]
            n205 = Initialize Array(0, w316) -> (w315:i32[])
            n206 = property on="Listbox" class="LstBox (strict)"("Top Row"=w314, "Value"=w314, "Item Symbols"=w315) -> ()  [unwired: 2 in, 2 out]
          }
        }
      }
      event "Listbox": Key Down {
        # "Update symbols on the listbox\nLeft and right keys check and uncheck"
        n207 = event-data() -> ("VKey"=w320:T20)  [unwired: 1 in]
        n208 = case shown="\"Left\", \"Right\"" w320 {
          selector: w320 -> [w325 _]
          tunnel: eventvkey."Left" ("VKey") -> [w323 _]
          frame "Left", "Right" {
            n209 = Equal?(x=w323, y=w325) -> (x = y?=w324:bool)
            n210 = Select(t=0, s=w324, f=1) -> (s? t:f=w326:i32)
            n211 = property on="Listbox" class="LstBox (strict)"() -> ("Item Symbols"=w329:i32[])  [unwired: 2 in, 2 out]
            n212 = Replace Array Subset(array=w329, new element=w326, index="Listbox") -> (w328:i32[])
            n213 = property on="Listbox" class="LstBox (strict)"("Item Symbols"=w328) -> ()  [unwired: 2 in, 2 out]
          }
          frame Default {
          }
        }
      }
      event "DB Camera Config": Value Change {
        # "Show or hide the cluster of controls, store in ini file"
        n214 = event-data() -> ("NewVal"=w333:bool)  [unwired: 1 in]
        n215 = case shown="False" w333 {
          tunnel: w332 -> [w342 _]
          tunnel: [w335 w353] -> w331
          tunnel: w330 -> [w334 w353]
          frame False {
            w349 = "Camera"
            w352 = FALSE ("Visible")
            n216 = local read "Camera Settings"() -> (w341:T2)
            n217 = Index Array(array=w342) -> (element=w345:cluster{string[]})  [unwired: 1 in]
            n218 = Unbundle(w341) -> ("Frame Rate"=w340:i32, "Compression"=w339:i32, "Size"=w343:u16)
            n219 = Unbundle(w345) -> (w344:string[])
            n220 = Index Array(array=w344, index=w343) -> (element=w338:string)
            n221 = call-poly <vilib>:"Write Key.vi"("section"=w349, "value"=w338, "key"="Size", "refnum"=w334) -> ("refnum out"=w351:T18)  [unwired: 2 in, 5 out]
            n222 = call-poly <vilib>:"Write Key.vi"("section"=w349, "value"=w340, "key"="FrameRate", "refnum"=w351) -> ("refnum out"=w350:T18)  [unwired: 1 in, 6 out]
            n223 = property on="Camera Settings" class="Clust (strict)"("Visible"=w352) -> ()  [unwired: 2 in, 2 out]
            n224 = local write "DB Camera Config"(w352) -> ()
            n225 = call-poly <vilib>:"Write Key.vi"("section"=w349, "value"=w339, "key"="Compression", "refnum"=w350) -> ("refnum out"=w336:T18)  [unwired: 1 in, 6 out]
            n226 = call <vilib>:"Close Config Data.vi"("refnum"=w336) -> ("file path"=w337:path)  [unwired: 2 in, 8 out]
            n227 = call <vilib>:"Open Config Data.vi"("configuration file path"=w337) -> ("refnum"=w335:T18)  [unwired: 8 in, 2 out]
          }
          frame True {
            n228 = property on="Camera Settings" class="Clust (strict)"("Visible"=TRUE) -> ()  [unwired: 2 in, 2 out]
          }
        }
      }
      event "Camera Settings": Value Change {
        # "Update summary string when any elements of DB camera change"
        n229 = event-data() -> ("NewVal"=w366:T2)  [unwired: 1 in]
        n230 = Index Array(array=w362) -> (element=w361:cluster{string[]})  [unwired: 1 in]
        n231 = Unbundle(w366) -> ("Frame Rate"=w357:i32, "Compression"=w356:i32, "Size"=w359:u16)
        n232 = Unbundle(w361) -> (w360:string[])
        n233 = Index Array(array=w360, index=w359) -> (element=w358:string)
        n234 = Format Into String(format string="%s   %dfps   %d%%", w358, w357, w356) -> (resulting string=w363:string)  [unwired: 2 in, 1 out]
        n235 = Build Array(w363) -> (w364:string[])
        n236 = property on="DB Camera Config" class="Bool (strict)"("Strings [4]"=w364) -> ()  [unwired: 2 in, 2 out]
      }
      event "Motor.Enable": Value Change {
        # "When the test mode otor enable helper is set, update that\ntree row item's value"
        n237 = event-data() -> ("NewVal"=w372:bool)  [unwired: 1 in]
        n238 = Unbundle("Motor") -> ("Value"=w371:dbl)  [unwired: 1 out]
        n239 = Select(t=w371, s=w372, f=0.0) -> (s? t:f=w369:dbl)
        n240 = call <vilib>:"NT Write Number.vi"("Numeric"=w369, "Name"=w368) -> ()  [unwired: 9 in, 1 out]
      }
      event "Test Slider": Value Change {
        # "When the test mode slider helper is set, update that\ntree row item's value"
        n241 = event-data() -> ("NewVal"=w375:dbl)  [unwired: 1 in]
        n242 = call <vilib>:"NT Write Number.vi"("Numeric"=w375, "Name"=w376) -> ()  [unwired: 9 in, 1 out]
      }
      event "On/Off": Value Change {
        # "When the test mode on/off helper value is set, update that\ntree row item's value"
        n243 = event-data() -> ("NewVal"=w380:bool)  [unwired: 1 in]
        n244 = Boolean To (0,1)(Boolean=w380) -> (0, 1=w379:i16)
        n245 = call <vilib>:"NT Write Number.vi"("Numeric"=w379, "Name"=w378) -> ()  [unwired: 9 in, 1 out]
      }
      event "Rev/Fwd": Value Change {
        # "When the test mode helper value for relays is set, update that\ntree row item's value"
        n246 = event-data() -> ("NewVal.Forward"=w388:bool, "NewVal.Reverse"=w387:bool)  [unwired: 1 in]
        n247 = Boolean To (0,1)(Boolean=w388) -> (0, 1=w384:i16)
        n248 = Boolean To (0,1)(Boolean=w387) -> (0, 1=w386:i16)
        n249 = Negate(x=w386) -> (-x=w385:i16)
        n250 = Add(x=w384, y=w385) -> (x+y=w383:i16)
        n251 = call <vilib>:"NT Write Number.vi"("Numeric"=w383, "Name"=w382) -> ()  [unwired: 9 in, 1 out]
      }
      event "Test Ring": Value Change {
        # "When a test mode helper value is selected from the ring,\nset the tree item's variable to the string value"
        n252 = event-data() -> ("NewVal"=w392:u16)  [unwired: 1 in]
        n253 = property on="Test Ring" class="Ring (strict)"() -> ("Strings []"=w393:string[])  [unwired: 2 in, 2 out]
        n254 = Index Array(array=w393, index=w392) -> (element=w391:string)
        n255 = call <vilib>:"NT Write String.vi"("String"=w391, "Name"=w390) -> ()  [unwired: 9 in, 1 out]
      }
      event "Rec Mode": Value Change {
        # "Update globals for recording mode and path to read log from.\nClear when logging and let NetworkTables set path for vision to\nuse."
        n256 = event-data() -> ("NewVal"=w403:enum32{"Stop", "Record", "Playback"})  [unwired: 1 in]
        n257 = global write "WPI_DashboardLogging Global.vi" "Logging Filename"(path "") -> ()
        n258 = case shown="\"Playback\"" w403 {
          tunnel: w402 -> [_ w405 w413]
          tunnel: [_ _ w412] -> w399
          tunnel: [_ _ w411] -> _
          tunnel: w397 -> [_ _ w409]
          tunnel: cluster{i32, i32} {-250, 170} -> [_ _ w408]
          tunnel: [_ _ T21 {"Image Size"=TRUE, "Image Type"=TRUE, "Pixel Value"=TRUE, "ROI Information"=TRUE, "Zoom Factor"=FALSE} ("Image Information Shown:All Elements")] -> w395
          tunnel: [_ _ TRUE ("Zoom Factor")] -> w394
          frame Default {
          }
          frame "Stop", "Record" {
            # "Place Window too"
            n259 = invoke class="VI" method="FP.Close"(reference=w405) -> (reference out=w404:refnum<vi>)  [unwired: 2 in, 2 out]
            n260 = invoke class="VI" method="Abort VI"(reference=w404) -> ()  [unwired: 2 in, 3 out]
          }
          frame "Playback" {
            n261 = call "Open Playback Panel.vi"("Offset"=w408, "DB VI Ref"=w409, "Playback in"=w413) -> ("Playback out"=w410:refnum<vi>)  [unwired: 8 in]
            n262 = register-events(w410) -> (reference out=w412:refnum<event-registration>, error out=w411:errorcluster)  [unwired: 2 in]
          }
        }
        n263 = global write "WPI_DashboardLogging Global.vi" "Recording"(w403) -> ()
        n264 = property on="Camera Image" class="ImageControl"("Image Information Shown"=w395, "Image Information Visible"=w394) -> ()  [unwired: 2 in, 2 out]
        n265 = call <vilib>:"WPI_DashboardNT Log FieldName Cache.vi"("Operation"=enum16{"Lookup/Add", "Index", "Clear"}."Clear") -> ()  [unwired: 8 in, 3 out]
      }
      event Panel Close {
        w414 = enum32{"Stop", "Record", "Playback"}."Stop" ("Rec Mode")
        # "Playback window has been closed, abort"
        n266 = event-data() -> ()  [unwired: 1 in, 4 out]
        n267 = local write "Rec Mode"(w414) -> ()
        n268 = global write "WPI_DashboardLogging Global.vi" "Recording"(w414) -> ()
      }
      event Panel Close {
        # "Abort playback window and ourself"
        n269 = event-data() -> ()  [unwired: 1 in, 4 out]
        n270 = invoke class="VI" method="FP.Close"(reference=w419) -> (reference out=w418:refnum<vi>)  [unwired: 2 in, 2 out]
        n271 = invoke class="VI" method="Abort VI"(reference=w418) -> (error out=w417:errorcluster)  [unwired: 2 in, 2 out]
        n272 = invoke class="VI" method="Abort VI"(error in=w417) -> ()  [unwired: 2 in, 3 out]
      }
      event "Vision": Value Change {
        # "Enable/Disable Compression slider.\nHW USB is hard-coded into the camera"
        n273 = event-data() -> ("NewVal"=w425:u16)  [unwired: 1 in]
        n274 = Equal?(x=w425, y=u32 2 ("milliseconds to wait")) -> (x = y?=w423:bool)
        n275 = Select(t=T22."Disabled and Grayed Out" ("Disabled"), s=w423, f=T22."Enabled" ("Disabled")) -> (s? t:f=w420:T22)
        n276 = property on="Compression" class="Slide (strict)"("DisabledEnum"=w420) -> ()  [unwired: 2 in, 2 out]
      }
    }
  }
  n277 = while {
    tunnel: w38 -> [w428]
    i -> [w431]
    stop <- FALSE stop-if-true
    n278 = Wait (ms)(milliseconds to wait=u32 100) -> ()  [unwired: 1 out]
    n279 = case shown="\"Playback\"" "Rec Mode" {
      tunnel: w431 -> [_ _ w446]
      tunnel: [u32 2829099 ("Base Color") u32 11141120 ("Target Color") w435] -> w427
      frame "Stop", Default {
        # "Reset the color, extra updates don't cost much"
      }
      frame "Record" {
      }
      frame "Playback" {
        # "Playback"
        n280 = Quotient & Remainder(x=w446, y=u32 50 ("milliseconds to wait")) -> (x-y*floor(x/y)=w442:u32)  [unwired: 1 out]
        n281 = Divide(x=w442, y=u32 50 ("milliseconds to wait")) -> (x/y=w439:dbl)
        n282 = Multiply(x=6.283185307179586, y=w439) -> (x*y=w444:dbl)
        n283 = Sine(x=w444) -> (sin(x)=w443:dbl)
        n284 = Absolute Value(x=w443) -> (abs(x)=w436:dbl)
        n285 = call "Interpolate RGB Color.vi"("Proportion"=w436, "Target Color"=u32 30976, "Base Color"=u32 2829099) -> ("Result Color"=w435:u32)  [unwired: 8 in]
      }
    }
    n286 = property class="Pane"(reference=w428, "PaneColor"=w427) -> ()  [unwired: 1 in, 2 out]
  }
  n287 = TCP Create Listener(10:u16 1741 ("timeout ms (25000)")) -> (3:w1:refnum<k5>)  [unwired: 4 in, 2 out]
  n288 = while {
    tunnel: w1 -> [w448]
    stop <- FALSE stop-if-true
    n289 = TCP Wait On Listener(11:w448) -> (4:w447:refnum<k5>)  [unwired: 3 in, 4 out]
    n290 = local write "TCP"(w447) -> ()
  }
  n291 = property on="On/Off" class="Bool (strict)"("Visible"=w6) -> ()  [unwired: 2 in, 2 out]
  n292 = property on="Motor" class="Clust (strict)"("Visible"=w6) -> ()  [unwired: 2 in, 2 out]
  n293 = property on="Progress" class="Clust (strict)"("Visible"=w6) -> ()  [unwired: 2 in, 2 out]
  n294 = property on="Test Ring" class="Ring (strict)"("Visible"=w6) -> ()  [unwired: 2 in, 2 out]
  n295 = property on="Rev/Fwd" class="Clust (strict)"("Visible"=w6) -> ()  [unwired: 2 in, 2 out]
  n296 = property on="Camera Settings" class="Clust (strict)"("Visible"=w6) -> ()  [unwired: 2 in, 2 out]
  n297 = local write "DB Camera Config"(w6) -> ()
  n298 = global write "WPI_DashboardLogging Global.vi" "Recording"(w32) -> ()
  n299 = local write "Rec Mode"(w32) -> ()
